vi "PCIeDiffractiveTest.vi"() -> ()   [LabVIEW 2010]
uses:
  <vilib>/Utility/file.llb/Write To Spreadsheet File (I64).vi
  Blink_C_wrapper.dll
  ImageGen.dll
panel:
  out "Array":u8[][](array[numeric])
  out "BoardNum":i32
  # "PCIe  LabVIEWSDK"
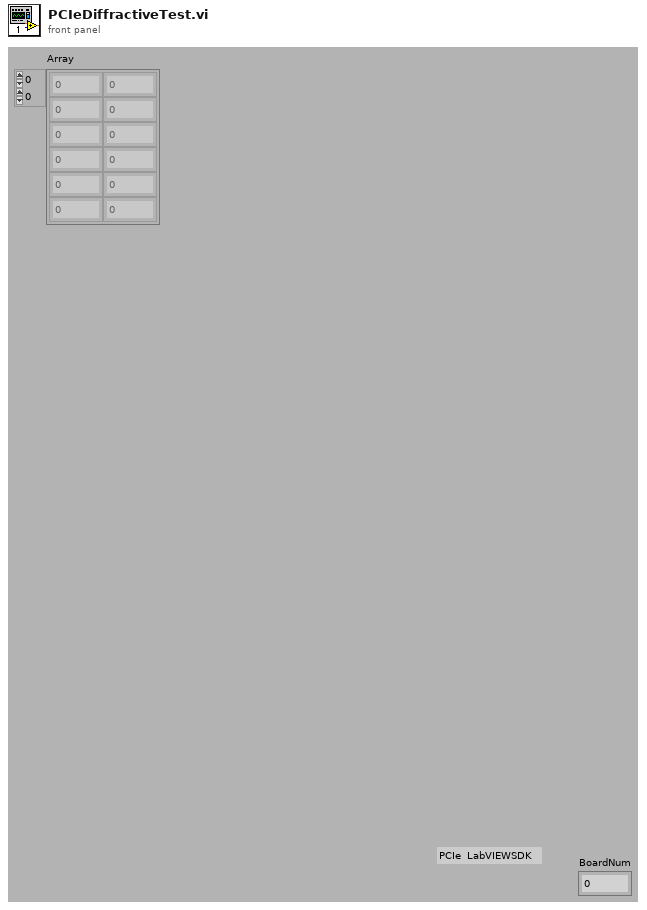
[diagram p1: front panel]
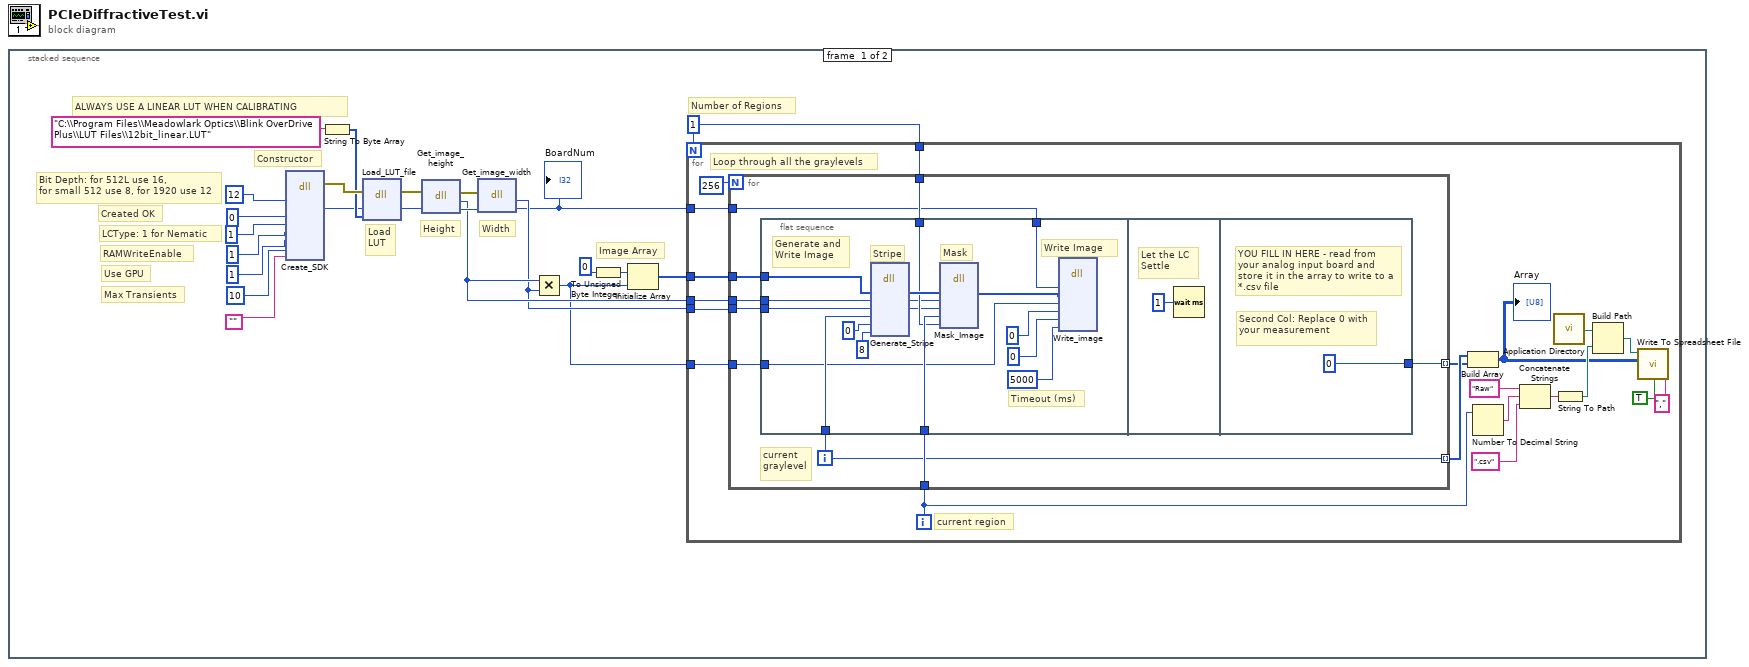
[diagram p0: block diagram]
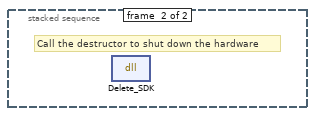
[diagram p2: hidden frame]
diagram:
  n1 = stacked-sequence {
    frame #0 {
      w5 = 1
      # "Number of Regions"
      # "Image Array"
      # "Width"
      # "Height"
      # "ALWAYS USE A LINEAR LUT WHEN CALIBRATING"
      # "Load\nLUT"
      # "Created OK"
      # "Max Transients"
      # "Use GPU"
      # "RAMWriteEnable"
      # "Bit Depth: for 512L use 16, \nfor small 512 use 8, for 1920 use 12"
      # "LCType: 1 for Nematic"
      # "Constructor"
      n2 = dll-call lib="C:/Meadowlark/Repos/overdrive-plus/src/Blink_SDK_example_grizzly/Blink_C_wrapper.dll" fn="Create_SDK"("SLM_bit_depth"=12, "constructed_ok"=0, "is_nematic_type"=1, "RAM_write_enable"=1, "use_GPU_if_available"=1, "max_transient_frames"=10, "static_regional_lut_file"="") -> (error out=w18:errorcluster, "n_boards_found"=w13:u64)  [unwired: 12 in, 1 out]
      n3 = String To Byte Array(string="C:\\Program Files\\Meadowlark Optics\\Blink OverDrive Plus\\LUT Files\\12bit_linear.LUT") -> (unsigned byte array=w17:u8[])
      n4 = dll-call lib="C:/Meadowlark/Repos/overdrive-plus/src/Blink_SDK_example_grizzly/Blink_C_wrapper.dll" fn="Load_LUT_file"(error in=w18, "Board"=w13, "LUTPath"=w17) -> (error out=w10:errorcluster, "Board"=w12:u32)  [unwired: 4 in, 1 out]
      n5 = dll-call lib="C:/Meadowlark/Repos/overdrive-plus/src/Blink_SDK_example_grizzly/Blink_C_wrapper.dll" fn="Get_image_height"(error in=w10, "Board"=w12) -> (error out=w9:errorcluster, "return type"=w4:i32, "Board"=w11:u32)  [unwired: 2 in, 1 out]
      n6 = dll-call lib="C:/Meadowlark/Repos/overdrive-plus/src/Blink_SDK_example_grizzly/Blink_C_wrapper.dll" fn="Get_image_width"(error in=w9, "Board"=w11) -> ("return type"=w3:i32, "Board"=w1:u32)  [unwired: 2 in, 2 out]
      "BoardNum" <- w1
      n7 = Multiply(x=w4, y=w3) -> (x*y=w2:i32)
      n8 = To Unsigned Byte Integer(number=0) -> (unsigned 8bit integer=w8:u8)
      n9 = Initialize Array(w8, w2) -> (w6:u8[])
      n10 = for {
        N: w5 -> [_]
        tunnel: w6 -> [w43]
        tunnel: w4 -> [w42]
        tunnel: w3 -> [w41]
        tunnel: w5 -> [w39]
        tunnel: w2 -> [w25]
        tunnel: w1 -> [w24]
        i -> [w37]
        # "current region"
        # "Loop through all the graylevels"
        n11 = for {
          N: 256 -> [_]
          tunnel: w43 -> [w52]
          tunnel: w42 -> [w51]
          tunnel: w41 -> [w50]
          tunnel: w37 -> [w49]
          tunnel: w39 -> [w48]
          tunnel: [w47] -> w27 mode=indexing
          tunnel: [w46] -> w26 mode=indexing
          tunnel: w25 -> [w45]
          tunnel: w24 -> [w44]
          i -> [w47]
          # "current \ngraylevel"
          n12 = flat-sequence {
            tunnel: w52 -> [w69]
            tunnel: w51 -> [w66]
            tunnel: w50 -> [w65]
            tunnel: w49 -> [w64]
            tunnel: w48 -> [w63]
            tunnel: w47 -> [w59]
            tunnel: w45 -> [w54]
            tunnel: w44 -> [w53]
            tunnel: [0] -> w46
            frame #0 {
              # "Timeout (ms)"
              # "Write Image"
              # "Generate and \nWrite Image"
              # "Mask"
              # "Stripe"
              n13 = dll-call lib="C:/Meadowlark/Repos/overdrive-plus/src/Blink_SDK_example_grizzly/ImageGen.dll" fn="Generate_Stripe"("Array"=w69, "Width"=w66, "Height"=w65, "PixelValOne"=w59, "PixelValTwo"=0, "PixelsPerStripe"=8) -> ("Array"=w67:u8[], "Width"=w61:i32, "Height"=w62:i32)  [unwired: 7 in, 2 out]
              n14 = dll-call lib="C:/Meadowlark/Repos/overdrive-plus/src/Blink_SDK_example_grizzly/ImageGen.dll" fn="Mask_Image"("Array"=w67, "Width"=w61, "Height"=w62, "Region"=w64, "NumRegions"=w63) -> ("Array"=w55:u8[])  [unwired: 8 in, 2 out]
              n15 = dll-call lib="C:/Meadowlark/Repos/overdrive-plus/src/Blink_SDK_example_grizzly/Blink_C_wrapper.dll" fn="Write_image"("board"=w53, "Image"=w55, "ImageSize"=w54, "WaitForTrigger"=0, "ExternalPulse"=0, "timeout"=5000) -> ()  [unwired: 10 in, 2 out]
            }
            frame #1 {
              # "Let the LC \nSettle"
              n16 = Wait (ms)(milliseconds to wait=u32 1) -> ()  [unwired: 1 out]
            }
            frame #2 {
              # "Second Col: Replace 0 with your measurement"
              # "YOU FILL IN HERE - read from  your analog input board and store it in the array to write to a *.csv file"
            }
          }
        }
        n17 = Build Array(w27, w26) -> (w28:i32[][])
        "Array" <- w28
        n18 = Number To Decimal String(number=w37) -> (decimal integer string=w36:string)  [unwired: 1 in]
        n19 = Concatenate Strings("Raw", w36, ".csv") -> (w34:string)
        n20 = call <vilib>:"Application Directory.vi"() -> ("Application Directory"=w33:path)
        n21 = String To Path(string=w34) -> (path=w32:path)
        n22 = Build Path(base path=w33, name or relative path=w32) -> (appended path=w31:path)
        n23 = call-poly <vilib>:"Write To Spreadsheet File.vi"("delimiter (\\t)"=",", "transpose? (no:F)"=TRUE, "2D data"=w28, "file path (dialog if empty)"=w31) -> ()  [unwired: 4 in, 1 out]
      }
    }
    frame #1 {
      # "Call the destructor to shut down the hardware"
      n24 = dll-call lib="C:/Meadowlark/Repos/overdrive-plus/src/Blink_SDK_example_grizzly/Blink_C_wrapper.dll" fn="Delete_SDK"() -> ()  [unwired: 4 in, 2 out]
    }
  }
